vi "Init.vi"(8 "error in (no error)":errorcluster) -> (0 "error out":errorcluster, 3 "View out":refnum<class "View.lvclass">)   [LabVIEW 2020, in "Page2.lvlib" / "View.lvclass"]
uses:
  View.lvclass
  View.lvclass/View.ctl
  Controller/Controller.lvclass
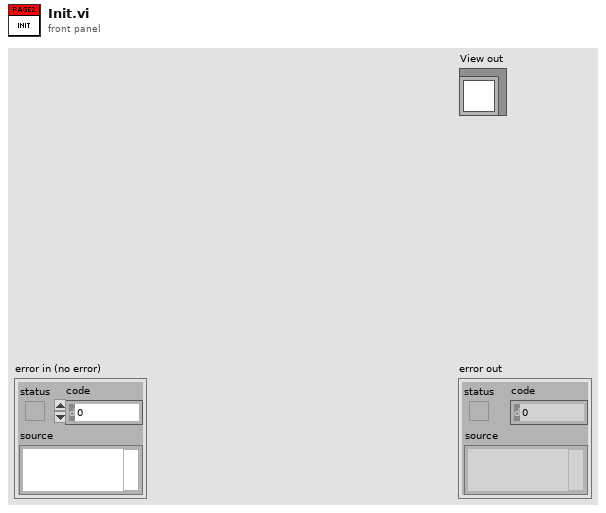
[diagram p1: front panel]
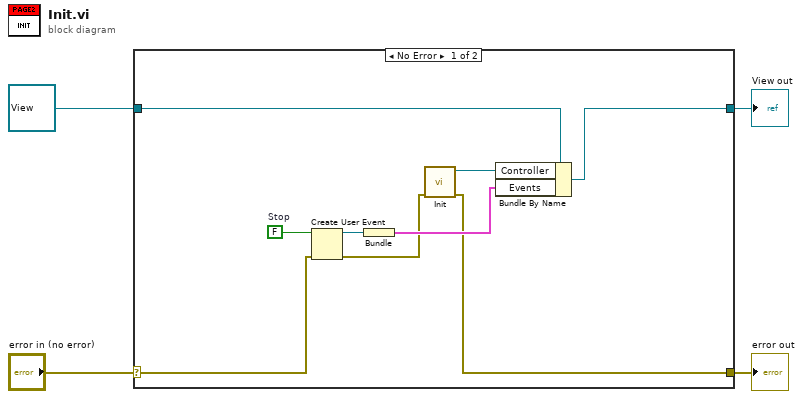
[diagram p0: block diagram]
diagram:
  n1 = case shown="No Error" "error in (no error)" {
    selector: "error in (no error)" -> [w8 w15]
    tunnel: [w6 w15] -> w3
    tunnel: [w9 w14] -> w2
    tunnel: refnum<class "View.lvclass"> refnum ("View in") -> [w10 w14]
    frame No Error {
      w13 = FALSE  # Stop
      n2 = Create User Event(user event datatype=w13, error in=w8) -> (user event=w12:refnum<user-event>, error out=w7:errorcluster)
      n3 = Bundle("Stop"=w12) -> (w11:cluster{"Stop":refnum<user-event>})  [unwired: 1 in]
      n4 = call "Init.vi"("error in (no error)"=w7) -> ("error out"=w6:errorcluster, "Controller out"=w5:refnum<class "Controller.lvclass">)  [unwired: 9 in]
      n5 = Bundle By Name(cluster=w10, "Controller"=w5, "Events"=w11) -> (w9:refnum<class "View.lvclass">)
    }
    frame Error {
    }
  }
  "error out" <- w3
  "View out" <- w2
